vi "Actor Core.vi"(8 "error in":errorcluster, 11 "Async Actor Example in":refnum<class "Async Methods Actor Example.lvclass">) -> (0 "error out":errorcluster, 3 "Actor out":refnum<class "Actor.lvclass">)   [LabVIEW 2023, in "Async Methods Actor Example.lvlib" / "Async Methods Actor Example.lvclass"]
doc: "(<B>Filename</B>: Actor Framework.lvlib:Actor.lvclass:Actor Core.vi)\n\nReceives messages to the actor, reacts to them, and initiates any error handling that may shut the actor down.\n\nDescendant classes may override this VI to append parallel tasks for the actor to complete while it handles messages. Overrides use the Call Parent Class Method node."
uses:
  Async Methods Actor Example.lvclass
  C:/Program Files/National Instruments/LabVIEW 2023/vi.lib/ActorFramework/Actor/Actor.lvclass
  C:/Program Files/National Instruments/LabVIEW 2023/vi.lib/LS Instruments AG/Async Methods Actor/Async Methods Actor/Async Methods Actor/Async Methods Actor.lvclass
  <vilib>/ActorFramework/Actor/Actor.lvclass
  <vilib>/LS Instruments AG/Async Methods Actor/Async Methods Actor/Async Methods Actor/Async Call Method.ctl
  <vilib>/LS Instruments AG/Async Methods Actor/Async Methods Actor/Async Methods Actor/Async Methods Running.ctl
  <vilib>/LS Instruments AG/Async Methods Actor/Async Methods Actor/Async Methods Actor/VI Refnum Lifetime.ctl
  <vilib>/ActorFramework/Actor/Actor.lvclass/Actor.ctl
  <vilib>/ActorFramework/Message Enqueuer/Message Enqueuer.lvclass/Message Enqueuer.ctl
  Async Methods Actor Example.lvclass/Async Methods Actor Example.ctl
  <vilib>/LS Instruments AG/Async Methods Actor/Async Methods Actor/Async Methods Actor/Async Methods Actor.lvclass/Async Methods Actor.ctl
  <vilib>/LS Instruments AG/Async Methods Actor/Async Methods Actor/Async Methods Actor Messages/Write Kill Methods On Exit Msg/Write Kill Methods On Exit Msg.lvclass/Write Kill Methods On Exit Msg.ctl
  <vilib>/LS Instruments AG/Async Methods Actor/Async Methods Actor/Async Methods Actor Messages/Async Message/Async Message.lvclass/Async Message.ctl
  Async Methods Actor Example Messages/Ack Completion Long Exec Meth Msg/Ack Completion Long Exec Meth Msg.lvclass
  C:/Program Files/National Instruments/LabVIEW 2023/vi.lib/LS Instruments AG/Async Methods Actor/Async Methods Actor/Async Methods Actor Messages/Completion Notification Msg/Completion Notification Msg.lvclass
  <vilib>/LS Instruments AG/Async Methods Actor/Async Methods Actor/Async Methods Actor Messages/Async Message/Async Message Settings.ctl
  <vilib>/ActorFramework/Message Enqueuer/Message Priority.ctl
  <vilib>/ActorFramework/Message Enqueuer/Message Enqueuer.lvclass
  <vilib>/LS Instruments AG/Async Methods Actor/Async Methods Actor/Async Methods Actor Messages/Completion Notification Msg/Completion Notification Msg.lvclass
  Async Methods Actor Example Messages/Ack Completion with Error Msg/Ack Completion with Error Msg.lvclass
  <vilib>/LS Instruments AG/Async Methods Actor/Async Methods Actor/Async Methods Actor Messages/Async Message/Read FQN.vi
  <vilib>/LS Instruments AG/Async Methods Actor/Async Methods Actor/Async Methods Actor Messages/Async Message/Read GUID.vi
  Read Completion Notification Data.vi
  <vilib>/LS Instruments AG/Async Methods Actor/Async Methods Actor/Async Methods Actor/Read Async Methods Running Event Ref.vi
  <vilib>/ActorFramework/Message Enqueuer/Init from Existing Queue.vi
  <vilib>/ActorFramework/Message Enqueuer/Enqueue.vi
  <vilib>/LS Instruments AG/Async Methods Actor/Async Methods Actor/Async Methods Actor/Get VI FQN.vi
  Async Methods Actor Example Messages/Cancel Long Exec Meth Msg/Cancel Long Exec Meth Msg.lvclass
  C:/Program Files/National Instruments/LabVIEW 2023/vi.lib/ActorFramework/Message/Message.lvclass
  <vilib>/LS Instruments AG/Async Methods Actor/Async Methods Actor/Async Methods Actor Messages/Write Kill Methods On Exit Msg/Write Kill Methods On Exit Msg.lvclass
  <vilib>/ActorFramework/Stop Msg/Stop Msg.lvclass
  <vilib>/ActorFramework/Message Priority Queue/Priority Enqueue.vi
  <vilib>/Utility/LVClass/Get LV Class Path.vi
  <vilib>/LS Instruments AG/Async Methods Actor/Async Methods Actor/Async Methods Actor/Async Methods Actor.lvclass
  <vilib>/LS Instruments AG/Async Methods Actor/Async Methods Actor/Async Methods Actor Messages/Async Message/Async Message.lvclass
  Async Methods Actor Example Messages/Alternative Long Execution Method Msg/Alternative Long Execution Method Msg.lvclass
  Async Methods Actor Example Messages/Error Reporting Test Msg/Error Reporting Test Msg.lvclass
  Async Methods Actor Example Messages/VI Refnum Lifetime Test Msg/VI Refnum Lifetime Test Msg.lvclass
  Async Methods Actor Example Messages/Long Execution Method Msg/Long Execution Method Msg.lvclass
panel:
  in  "Error Propagation Test Async Call Method":T1 caption="Async Call Method"
  in  "Start Error Propagation Test":bool
  in  "Error Test Test Async Call Method":T1 caption="Async Call Method"
  in  "Start Error Reporting Test":bool
  in  "VI Renum Lifetime Test Async Call Method":T1 caption="Async Call Method"
  in  "Start VI Refnum Lifetime Test":bool
  in  "VI Refnum Lifetime":T2
  out "Last Sent Async Message GUID":string
  out "Completion Log":string[][](table)
  in  "Start Alternative":bool
  out "Async Methods Running":T3
  in  "Kill Methods On Exit":bool
  in  "Async Call Method":T1
  in  "Exit":bool
  in  "Start":bool
  in  "Cancel":bool
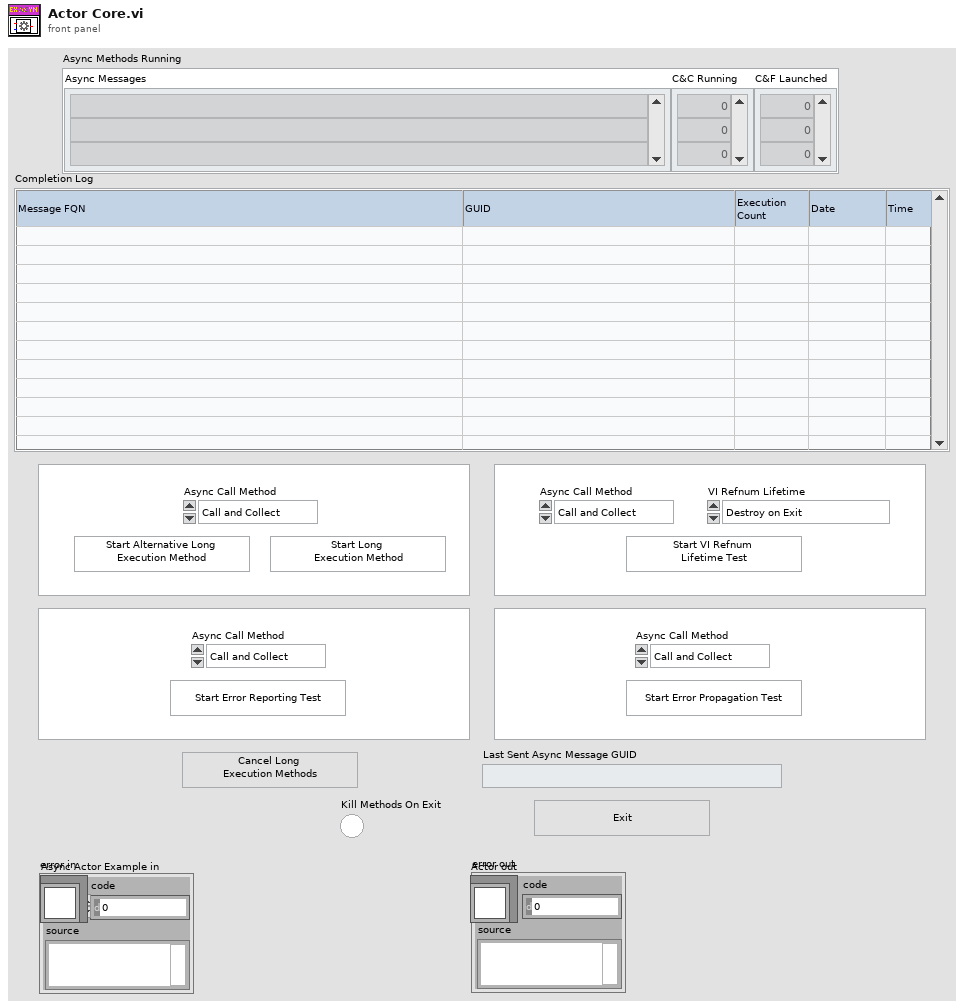
[diagram p1: front panel]
types:
  T1 = typedef "Async Methods Actor.lvlib/Async Methods Actor.lvclass/Async Call Method.ctl" = enum16{"Call and Collect", "Call and Forget"}
  T2 = typedef "Async Methods Actor.lvlib/Async Methods Actor.lvclass/VI Refnum Lifetime.ctl" = enum16{"Destroy on Exit", "Destroy on Actor Exit", "Destroy on Application Exit"}
  T3 = typedef "Async Methods Actor.lvlib/Async Methods Actor.lvclass/Async Methods Running.ctl" = cluster{"Async Messages":string[], "C&C Running":u32[], "C&F Launched":u32[]}
  T4 = enum8{"Enabled", "Disabled", "Disabled and Grayed Out"}
  T5 = typedef "Async Methods Actor.lvlib/Async Message.lvclass/Async Message Settings.ctl" = cluster{"Message Priority (Normal)":T6, "Async Call Method (Call and Collect)":T1, "VI Refnum Lifetime (Destroy on Actor Exit)":T2, "Report Errors (T)":bool, "Caller Enqueuer":refnum<class "Message Enqueuer.lvclass">, "Completion Notification Msg":refnum<class "Completion Notification Msg.lvclass">}
  T6 = typedef "Actor Framework.lvlib/Message Enqueuer.lvclass/Message Priority.ctl" = enum16{"Low", "Normal", "High"}
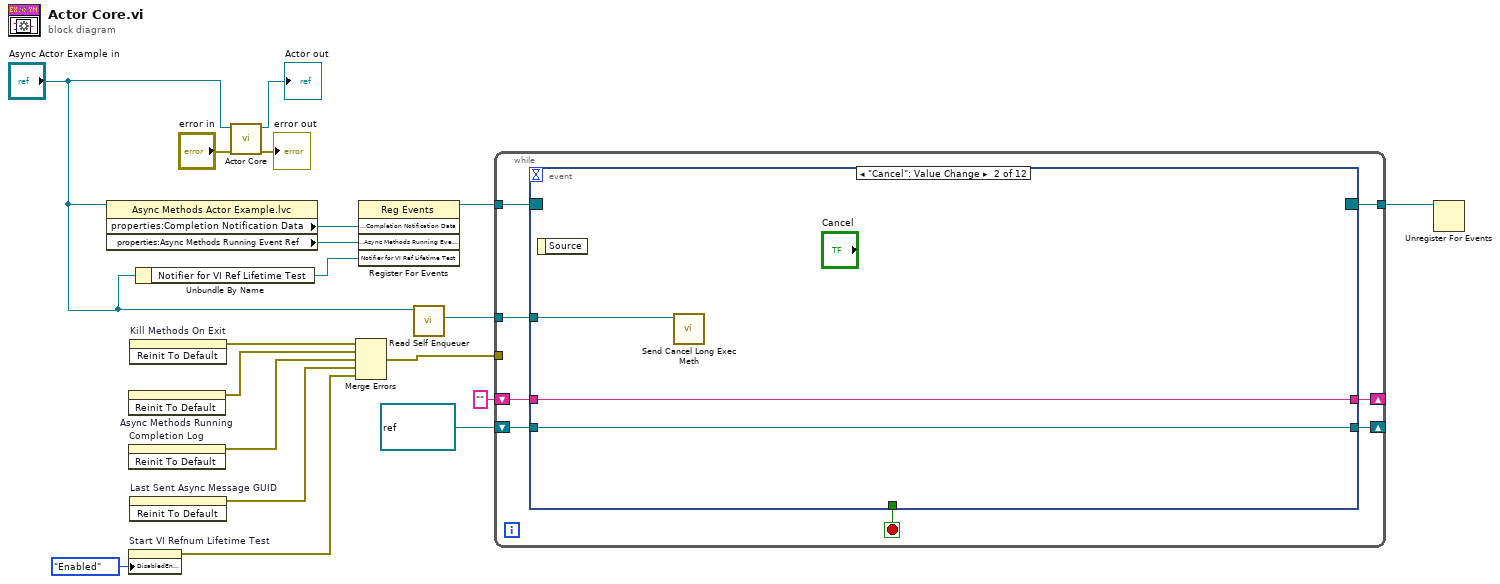
[diagram p0: block diagram]
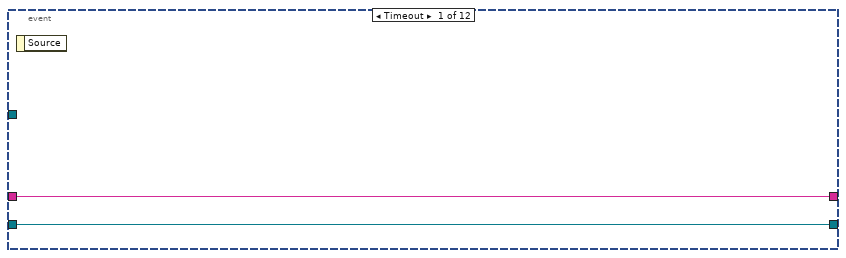
[diagram p2: hidden frame]
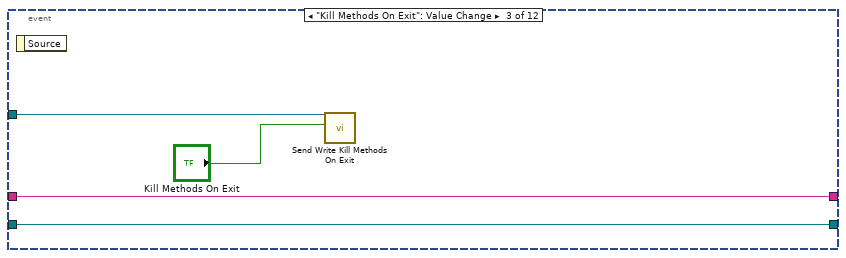
[diagram p3: hidden frame]
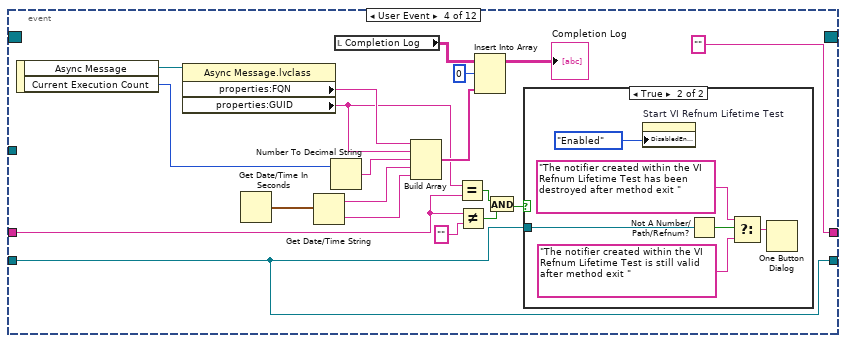
[diagram p4: hidden frame]
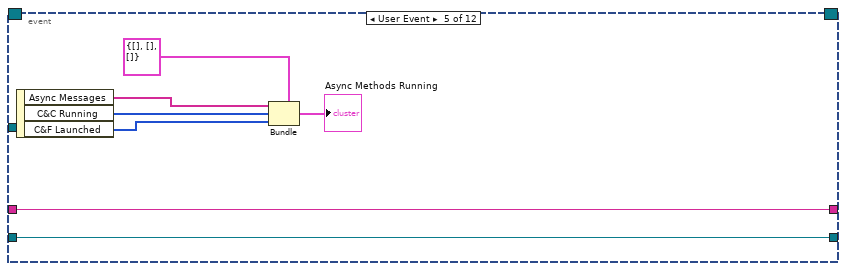
[diagram p6: hidden frame]
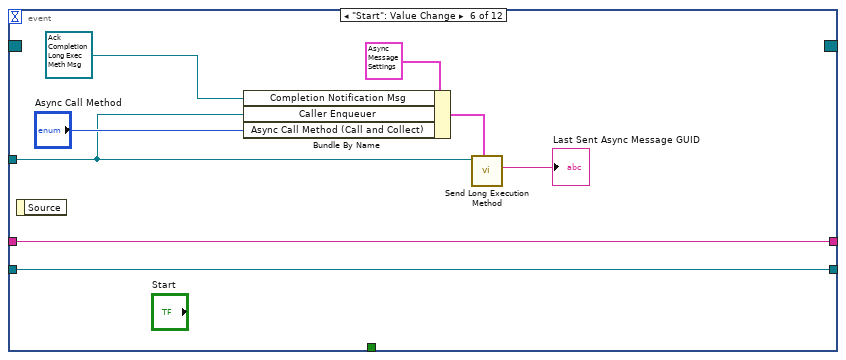
[diagram p7: hidden frame]
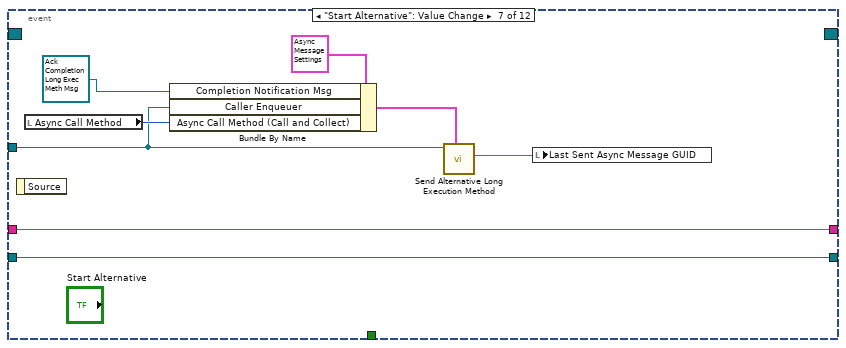
[diagram p8: hidden frame]
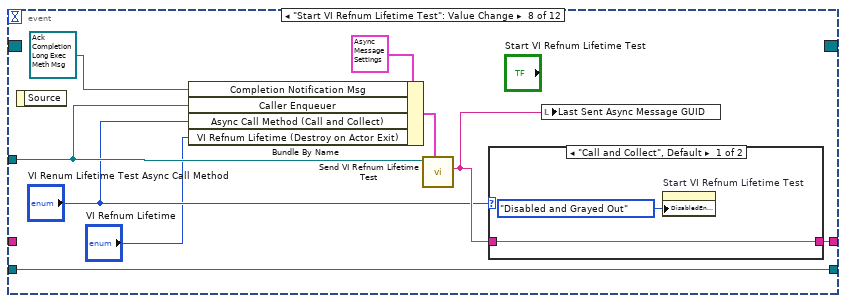
[diagram p9: hidden frame]
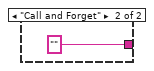
[diagram p10: hidden frame]
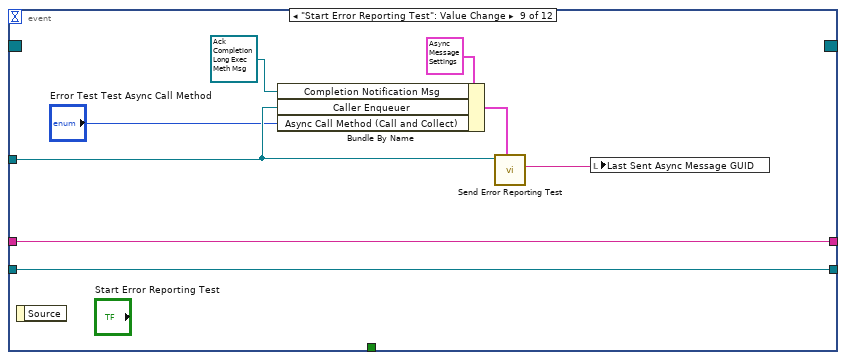
[diagram p11: hidden frame]
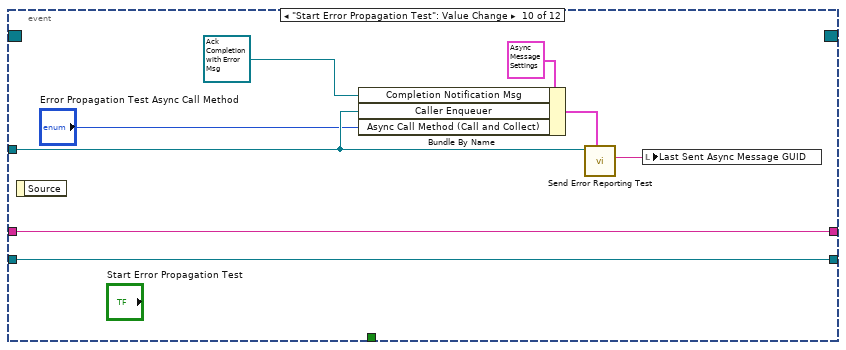
[diagram p12: hidden frame]
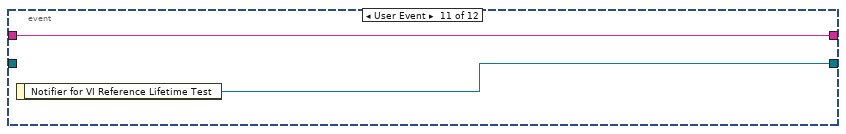
[diagram p13: hidden frame]
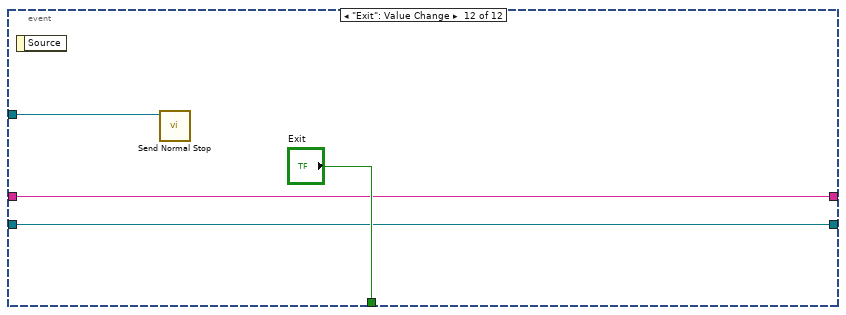
[diagram p14: hidden frame]
diagram:
  n1 = property class="Async Methods Actor Example.lvc"(reference="Async Actor Example in") -> ("properties:Completion Notification Data"=w14:refnum<user-event>, "properties:Async Methods Running Event Ref"=w11:refnum<user-event>)  [unwired: 1 in, 2 out]
  n2 = invoke on="Async Methods Running" class="Clust (strict)" method="Reinit To Default"() -> (error out=w9:errorcluster)  [unwired: 3 in, 2 out]
  n3 = invoke on="Completion Log" class="Tbl (strict)" method="Reinit To Default"() -> (error out=w8:errorcluster)  [unwired: 3 in, 2 out]
  n4 = property on="Start VI Refnum Lifetime Test" class="Bool"("DisabledEnum"=T4."Enabled" ("Disabled")) -> (error out=w4:errorcluster)  [unwired: 2 in, 1 out]
  n5 = invoke on="Kill Methods On Exit" class="Bool (strict)" method="Reinit To Default"() -> (error out=w15:errorcluster)  [unwired: 3 in, 2 out]
  n6 = invoke on="Last Sent Async Message GUID" class="Str" method="Reinit To Default"() -> (error out=w7:errorcluster)  [unwired: 3 in, 2 out]
  n7 = Unbundle By Name("Async Actor Example in") -> ("Notifier for VI Ref Lifetime Test"=w2:refnum<user-event>)
  n8 = call-parent "Actor Core.vi"("error in"="error in", "Actor in"="Async Actor Example in") -> ("error out"=→"error out":errorcluster, "Actor out"=→"Actor out":refnum<class "Actor.lvclass">)  [unwired: 8 in]
  n9 = Merge Errors(w15, w9, w8, w7, w4) -> (w10:errorcluster)
  n10 = register-events(w14, w11, w2) -> (reference out=w13:refnum<event-registration>)  [unwired: 2 in, 1 out]
  n11 = call <vilib>:"Read Self Enqueuer.vi"("Actor"="Async Actor Example in") -> ("Self Enqueuer"=w16:refnum<class "Message Enqueuer.lvclass">)  [unwired: 10 in]
  n12 = while {
    tunnel: w16 -> [w26]
    tunnel: w10 -> [_]
    tunnel: w13 -> [w25]
    tunnel: [w24] -> w12
    shift-right: [w23] -> _
    shift-left: "" ("GUID") -> [w22]
    shift-right: [w21] -> _
    shift-left: refnum<notifier> refnum ("Notifier for VI Reference Lifetime Test") -> [w20]
    stop <- w27 stop-if-true
    n13 = event shown="[1] \"Cancel\": Value Change" {
      selector: w25 -> [_ _ _ _ _ _ _ _ _ _ _ _]
      dyn-events: [_ _ _ _ _ _ _ _ _ _ _ _] -> w24
      timeout: _ -> [_ _ _ _ _ _ _ _ _ _ _ _]
      tunnel: [_ _ _ _ _ _ _ _ _ _ _ "Exit"] -> w27
      tunnel: w26 -> [w30 w33 w36 _ _ w71 w78 w88 w99 w107 _ w118]
      tunnel: [w30 _ _ _ _ _ _ _ _ _ _ _] -> _
      tunnel: [w29 w32 w35 "" ("GUID") w64 w77 w85 w93 w104 w112 w115 w117] -> w23
      tunnel: w22 -> [w29 w32 w35 w41 w64 w77 w85 _ w104 w112 w115 w117]
      tunnel: [w28 w31 w34 w39 w63 w76 w84 w94 w105 w113 w114 w116] -> w21
      tunnel: w20 -> [w28 w31 w34 w39 w63 w76 w84 w94 w105 w113 _ w116]
      event Timeout {
        n14 = event-data() -> ()  [unwired: 1 in, 1 out]
      }
      event "Cancel": Value Change {
        n15 = event-data() -> ()  [unwired: 1 in, 1 out]
        n16 = call "Send Cancel Long Exec Meth.vi"("Message Enqueuer"=w33) -> ()  [unwired: 9 in, 2 out]
      }
      event "Kill Methods On Exit": Value Change {
        n17 = event-data() -> ()  [unwired: 1 in, 1 out]
        n18 = call <vilib>:"Send Write Kill Methods On Exit.vi"("Kill Methods On Exit"="Kill Methods On Exit", "Message Enqueuer in"=w36) -> ()  [unwired: 8 in, 2 out]
      }
      event User Event {
        n19 = event-data() -> ("Async Message"=w47:refnum<class "Async Message.lvclass">, "Current Execution Count"=w56:u32)  [unwired: 1 in]
        n20 = property class="Async Message.lvclass"(reference=w47) -> ("properties:FQN"=w46:string, "properties:GUID"=w38:string)  [unwired: 1 in, 2 out]
        n21 = Get Date/Time In Seconds() -> (seconds since 1Jan1904=w54:timestamp)
        n22 = Get Date/Time String(seconds (now)=w54) -> (date string=w53:string, time string=w52:string)  [unwired: 2 in]
        n23 = Number To Decimal String(number=w56) -> (decimal integer string=w55:string)  [unwired: 1 in]
        n24 = local read "Completion Log"() -> (w51:string[][])
        n25 = Build Array(w46, w38, w55, w53, w52) -> (w49:string[])
        n26 = Equal?(x=w38, y=w41) -> (x = y?=w45:bool)
        n27 = Not Equal?(x=w41, y="" ("GUID")) -> (x != y?=w42:bool)
        n28 = Insert Into Array(array=w51, index (row)=0, new element=w49) -> (→"Completion Log":string[][])  [unwired: 1 in]
        n29 = And(x=w45, y=w42) -> (x .and. y?=w43:bool)
        n30 = case shown="True" w43 {
          tunnel: w39 -> [_ w61]
          frame False {
          }
          frame True {
            n31 = property on="Start VI Refnum Lifetime Test" class="Bool"("DisabledEnum"=T4."Enabled" ("Disabled")) -> ()  [unwired: 2 in, 2 out]
            n32 = Not A Number/Path/Refnum?(number/path/refnum=w61) -> (NaN/Path/Refnum?=w60:bool)
            n33 = Select(t="The notifier created within the VI Refnum Lifetime Test has been destroyed after method exit " ("GUID"), s=w60, f="The notifier created within the VI Refnum Lifetime Test is still valid after method exit " ("GUID")) -> (s? t:f=w59:string)
            n34 = One Button Dialog(message=w59) -> ()  [unwired: 1 in, 1 out]
          }
        }
      }
      event User Event {
        n35 = event-data() -> ("Async Messages"=w68:string[], "C&C Running"=w66:u32[], "C&F Launched"=w65:u32[])  [unwired: 1 in]
        n36 = Bundle(cluster=T3 {"Async Messages"=[], "C&C Running"=[], "C&F Launched"=[]} ("Async Methods Running"), "Async Messages"=w68, "C&C Running"=w66, "C&F Launched"=w65) -> (→"Async Methods Running":T3)
      }
      event "Start": Value Change {
        n37 = event-data() -> ()  [unwired: 1 in, 1 out]
        n38 = Bundle By Name(cluster=T5 {"Message Priority (Normal)"=enum."Normal", "Async Call Method (Call and Collect)"=enum."Call and Collect", "VI Refnum Lifetime (Destroy on Actor Exit)"=enum."Destroy on Actor Exit", "Report Errors (T)"=TRUE, "Caller Enqueuer"=refnum, "Completion Notification Msg"=refnum} ("Async Message Settings"), "Completion Notification Msg"=refnum<class "Ack Completion Long Exec Meth Msg.lvclass"> refnum ("Async Methods Actor Example.lvlib:Ack Completion Long Exec Meth Msg.lvclass"), "Caller Enqueuer"=w71, "Async Call Method (Call and Collect)"="Async Call Method") -> (w74:T5)
        n39 = call "Send Long Execution Method.vi"("Async Message Settings"=w74, "Message Enqueuer in"=w71) -> ("GUID"=→"Last Sent Async Message GUID":string)  [unwired: 7 in, 2 out]
      }
      event "Start Alternative": Value Change {
        n40 = event-data() -> ()  [unwired: 1 in, 1 out]
        n41 = local read "Async Call Method"() -> (w79:T1)
        n42 = Bundle By Name(cluster=T5 {"Message Priority (Normal)"=enum."Normal", "Async Call Method (Call and Collect)"=enum."Call and Collect", "VI Refnum Lifetime (Destroy on Actor Exit)"=enum."Destroy on Actor Exit", "Report Errors (T)"=TRUE, "Caller Enqueuer"=refnum, "Completion Notification Msg"=refnum} ("Async Message Settings"), "Completion Notification Msg"=refnum<class "Ack Completion Long Exec Meth Msg.lvclass"> refnum ("Async Methods Actor Example.lvlib:Ack Completion Long Exec Meth Msg.lvclass"), "Caller Enqueuer"=w78, "Async Call Method (Call and Collect)"=w79) -> (w82:T5)
        n43 = call "Send Alternative Long Execution Method.vi"("Async Message Settings"=w82, "Message Enqueuer in"=w78) -> ("GUID"=w81:string)  [unwired: 7 in, 2 out]
        n44 = local write "Last Sent Async Message GUID"(w81) -> ()
      }
      event "Start VI Refnum Lifetime Test": Value Change {
        n45 = event-data() -> ()  [unwired: 1 in, 1 out]
        n46 = Bundle By Name(cluster=T5 {"Message Priority (Normal)"=enum."Normal", "Async Call Method (Call and Collect)"=enum."Call and Collect", "VI Refnum Lifetime (Destroy on Actor Exit)"=enum."Destroy on Actor Exit", "Report Errors (T)"=TRUE, "Caller Enqueuer"=refnum, "Completion Notification Msg"=refnum} ("Async Message Settings"), "Completion Notification Msg"=refnum<class "Ack Completion Long Exec Meth Msg.lvclass"> refnum ("Async Methods Actor Example.lvlib:Ack Completion Long Exec Meth Msg.lvclass"), "Caller Enqueuer"=w88, "Async Call Method (Call and Collect)"="VI Renum Lifetime Test Async Call Method", "VI Refnum Lifetime (Destroy on Actor Exit)"="VI Refnum Lifetime") -> (w90:T5)
        n47 = call "Send VI Refnum Lifetime Test.vi"("Async Message Settings"=w90, "Message Enqueuer in"=w88) -> ("GUID"=w92:string)  [unwired: 7 in, 2 out]
        n48 = case shown="\"Call and Collect\", Default" "VI Renum Lifetime Test Async Call Method" {
          tunnel: w92 -> [w96 _]
          tunnel: [w96 "" ("GUID")] -> w93
          frame "Call and Collect", Default {
            n49 = property on="Start VI Refnum Lifetime Test" class="Bool"("DisabledEnum"=T4."Disabled and Grayed Out" ("Disabled")) -> ()  [unwired: 2 in, 2 out]
          }
          frame "Call and Forget" {
          }
        }
        n50 = local write "Last Sent Async Message GUID"(w92) -> ()
      }
      event "Start Error Reporting Test": Value Change {
        n51 = event-data() -> ()  [unwired: 1 in, 1 out]
        n52 = Bundle By Name(cluster=T5 {"Message Priority (Normal)"=enum."Normal", "Async Call Method (Call and Collect)"=enum."Call and Collect", "VI Refnum Lifetime (Destroy on Actor Exit)"=enum."Destroy on Actor Exit", "Report Errors (T)"=TRUE, "Caller Enqueuer"=refnum, "Completion Notification Msg"=refnum} ("Async Message Settings"), "Completion Notification Msg"=refnum<class "Ack Completion Long Exec Meth Msg.lvclass"> refnum ("Async Methods Actor Example.lvlib:Ack Completion Long Exec Meth Msg.lvclass"), "Caller Enqueuer"=w99, "Async Call Method (Call and Collect)"="Error Test Test Async Call Method") -> (w102:T5)
        n53 = call "Send Error Reporting Test.vi"("Async Message Settings"=w102, "Message Enqueuer in"=w99) -> ("GUID"=w101:string)  [unwired: 7 in, 2 out]
        n54 = local write "Last Sent Async Message GUID"(w101) -> ()
      }
      event "Start Error Propagation Test": Value Change {
        n55 = event-data() -> ()  [unwired: 1 in, 1 out]
        n56 = Bundle By Name(cluster=T5 {"Message Priority (Normal)"=enum."Normal", "Async Call Method (Call and Collect)"=enum."Call and Collect", "VI Refnum Lifetime (Destroy on Actor Exit)"=enum."Destroy on Actor Exit", "Report Errors (T)"=TRUE, "Caller Enqueuer"=refnum, "Completion Notification Msg"=refnum} ("Async Message Settings"), "Completion Notification Msg"=refnum<class "Ack Completion with Error Msg.lvclass"> refnum ("Async Methods Actor Example.lvlib:Ack Completion with Error Msg.lvclass"), "Caller Enqueuer"=w107, "Async Call Method (Call and Collect)"="Error Propagation Test Async Call Method") -> (w109:T5)
        n57 = call "Send Error Reporting Test.vi"("Async Message Settings"=w109, "Message Enqueuer in"=w107) -> ("GUID"=w111:string)  [unwired: 7 in, 2 out]
        n58 = local write "Last Sent Async Message GUID"(w111) -> ()
      }
      event User Event {
        n59 = event-data() -> ("Notifier for VI Reference Lifetime Test"=w114:refnum<notifier>)  [unwired: 1 in]
      }
      event "Exit": Value Change {
        n60 = event-data() -> ()  [unwired: 1 in, 1 out]
        n61 = call <vilib>:"Send Normal Stop.vi"("Message Enqueuer"=w118) -> ()  [unwired: 10 in, 1 out]
      }
    }
  }
  n62 = Unregister For Events(event registration refnum=w12) -> ()  [unwired: 1 in, 1 out]
